vi "子VI.vi"() -> (1 "output":i32)   [LabVIEW 2011]
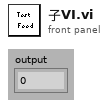
[diagram p1: front panel]
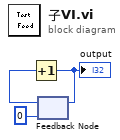
[diagram p0: block diagram]
diagram:
  n1 = feedback #1(0) -> (w2:i32)
  n2 = Increment(x=w2) -> (x+1=w1:i32)
  "output" <- w1
  n3 = feedback-in #1(w1) -> ()
